vi "update_position.vi"(8 "error in (no error)":errorcluster, 11 "DL090602SutterMP285Stage in":refnum<class "StageMMS2015ASI.lvclass">) -> (0 "error out":errorcluster, 3 "DL090602SutterMP285Stage out":refnum<class "StageMMS2015ASI.lvclass">)   [LabVIEW 2010, in "StageMMS2015ASI.lvclass"]
uses:
  StageMMS2015ASI.lvclass
  StageDL090409Scaffold/StageDL090409Scaffold/StageDL090409Scaffold.lvclass
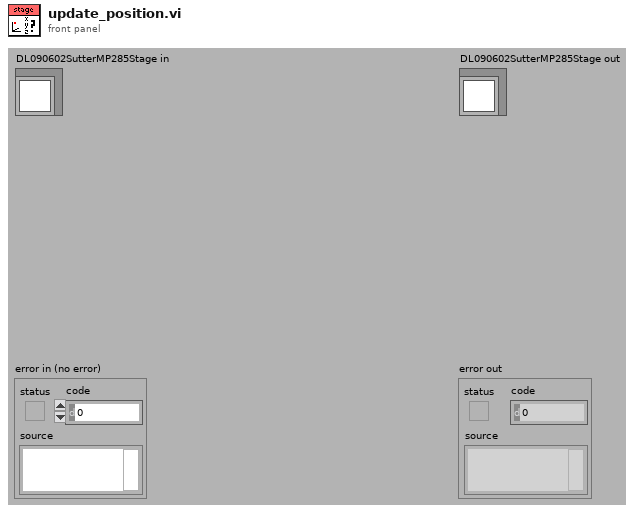
[diagram p1: front panel]
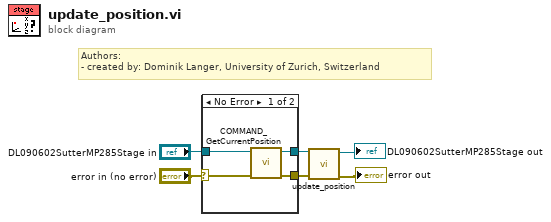
[diagram p0: block diagram]
diagram:
  # "Authors: \n- created by: Dominik Langer, University of Zurich, Switzerland"
  n1 = case shown="No Error" "error in (no error)" {
    selector: "error in (no error)" -> [w8 w12]
    tunnel: [w10 w12] -> w4
    tunnel: [w9 w11] -> w3
    tunnel: "DL090602SutterMP285Stage in" -> [w7 w11]
    frame No Error {
      n2 = call-dynamic "COMMAND_GetCurrentPosition.vi"("error in (no error)"=w8, "StageDL090602SutterMP285 in"=w7) -> ("error out"=w10:errorcluster, "StageDL090602SutterMP285 out"=w9:refnum<class "StageMMS2015ASI.lvclass">)  [unwired: 7 in, 1 out]
    }
    frame Error {
    }
  }
  n3 = call-parent "update_position.vi"("error in (no error)"=w4, "DL090409StageScaffold in"=w3) -> ("error out"=→"error out":errorcluster, "DL090409StageScaffold out"=→"DL090602SutterMP285Stage out":refnum<class "StageMMS2015ASI.lvclass">)  [unwired: 8 out]
